vi "ReadIO.fpga.vi"(10 "x (in)":u32, 11 "Memory In":refnum<k21>="InputMatrix") -> (2 "x (out)":u32)   [LabVIEW 2012]
uses:
  <vilib>/rvi/eio/common/nirviEmuTemplateMethod_errors.vi
  <vilib>/rvi/DataTransferAndStorage/Container/Common/niFpgaContainerExecOnDevCompGetState.vi
  <vilib>/rvi/DataTransferAndStorage/Container/Common/niFpgaContainerGetUniqueNameForEmu.vi
  <vilib>/rvi/Memory/Memory_Emulation/niFpgaMemoryEmulationCacheClearOnFirstRun.vi
  <vilib>/rvi/Memory/Memory_Emulation/nirvimemoryEmulationManagerCache_MakeExclusive.vi
  <vilib>/rvi/Memory/Memory_Emulation/niFpgaMemoryEmulationValidateCache.vi
  <vilib>/rvi/Memory/Memory_Emulation/nirvimemoryEmulationManagerCache_ReleaseExclusive.vi
  <vilib>/rvi/Memory/Memory_Emulation/nirvimemoryEmulationManagerCache_InsertValue.vi
  <vilib>/Utility/error.llb/Clear Errors.vi
  <vilib>/rvi/Emulation/niFpgaSctlEmulationGetInTimedLoop.vi
  <vilib>/rvi/Memory/Memory_Emulation/nirvimemoryEmulationManagerCache_GetValue.vi
  <vilib>/rvi/Memory/Memory_Emulation/nirvimemoryEmulationManagerCache_SetValue.vi
  <vilib>/rvi/Emulation/niFpgaSctlEmulationResourceMgr.vi
  <vilib>/eio/EIONode/EIONode.xnode
  <vilib>/rvi/DataTransferAndStorage/Container/XNode/niFpgaContainer.xnode
  <vilib>/rvi/Memory/Memory_Emulation/niFpgaMemoryEmulationRefIn.vi
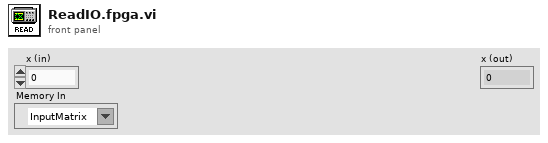
[diagram p1: front panel]
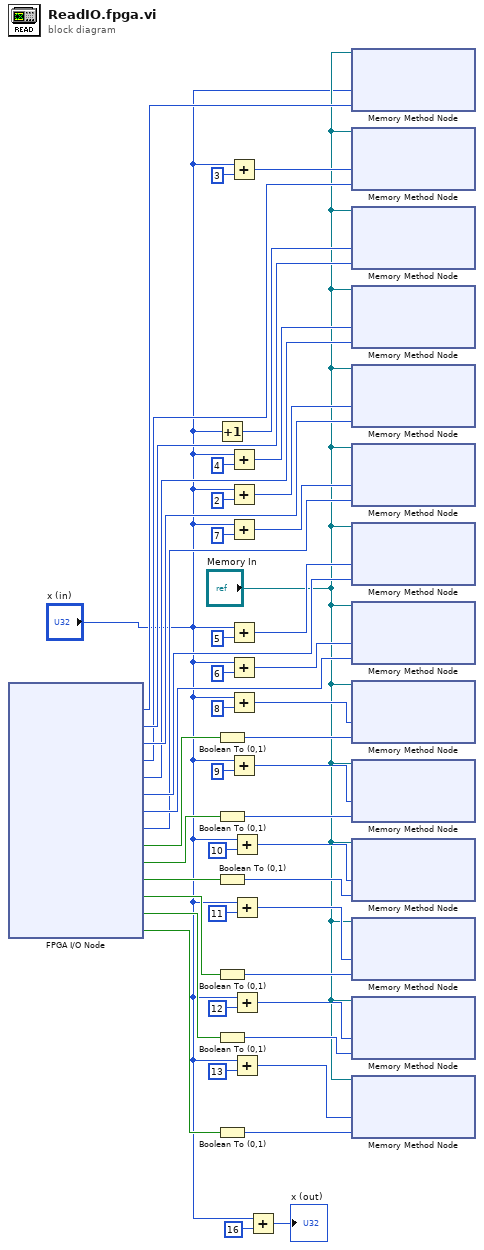
[diagram p0: block diagram]
diagram:
  n1 = xnode "FPGA I/O Node"() -> ("Connector0/AI0"=w49:i16, "Connector0/AI1"=w47:i16, "Connector0/AI2"=w46:i16, "Connector0/AI3"=w45:i16, "Connector0/AI4"=w44:i16, "Connector0/AI5"=w43:i16, "Connector0/AI6"=w42:i16, "Connector0/AI7"=w41:i16, "Connector0/DIO6"=w40:bool, "Connector0/DIO7"=w38:bool, "Connector0/DIO8"=w36:bool, "Connector0/DIO9"=w34:bool, "Connector0/DIO10"=w32:bool, "Connector0/DIO11"=w30:bool)  [unwired: 14 in, 14 out]
  n2 = Increment(x="x (in)") -> (x+1=w48:u32)
  n3 = Boolean To (0,1)(Boolean=w40) -> (0, 1=w39:i16)
  n4 = Boolean To (0,1)(Boolean=w38) -> (0, 1=w37:i16)
  n5 = Boolean To (0,1)(Boolean=w36) -> (0, 1=w35:i16)
  n6 = Boolean To (0,1)(Boolean=w34) -> (0, 1=w33:i16)
  n7 = Boolean To (0,1)(Boolean=w32) -> (0, 1=w31:i16)
  n8 = Boolean To (0,1)(Boolean=w30) -> (0, 1=w29:i16)
  n9 = Add(x="x (in)", y=u32 3) -> (x+y=w25:u32)
  n10 = Add(x="x (in)", y=u32 4) -> (x+y=w23:u32)
  n11 = Add(x="x (in)", y=u32 2) -> (x+y=w27:u32)
  n12 = Add(x="x (in)", y=u32 7) -> (x+y=w17:u32)
  n13 = Add(x="x (in)", y=u32 5) -> (x+y=w21:u32)
  n14 = Add(x="x (in)", y=u32 6) -> (x+y=w19:u32)
  n15 = Add(x="x (in)", y=u32 8) -> (x+y=w15:u32)
  n16 = Add(x="x (in)", y=u32 9) -> (x+y=w13:u32)
  n17 = Add(x="x (in)", y=u32 10) -> (x+y=w11:u32)
  n18 = Add(x="x (in)", y=u32 11) -> (x+y=w9:u32)
  n19 = Add(x="x (in)", y=u32 12) -> (x+y=w7:u32)
  n20 = Add(x="x (in)", y=u32 13) -> (x+y=w5:u32)
  n21 = Add(x="x (in)", y=u32 16) -> (x+y=→"x (out)":u32)
  n22 = xnode ("Memory Method Node")("Address"="x (in)", "Data"=w49, "Memory In"="Memory In") -> ()  [unwired: 1 out]
  n23 = xnode ("Memory Method Node")("Address"=w25, "Data"=w45, "Memory In"="Memory In") -> ()  [unwired: 1 out]
  n24 = xnode ("Memory Method Node")("Address"=w48, "Data"=w47, "Memory In"="Memory In") -> ()  [unwired: 1 out]
  n25 = xnode ("Memory Method Node")("Address"=w23, "Data"=w44, "Memory In"="Memory In") -> ()  [unwired: 1 out]
  n26 = xnode ("Memory Method Node")("Address"=w27, "Data"=w46, "Memory In"="Memory In") -> ()  [unwired: 1 out]
  n27 = xnode ("Memory Method Node")("Address"=w17, "Data"=w41, "Memory In"="Memory In") -> ()  [unwired: 1 out]
  n28 = xnode ("Memory Method Node")("Address"=w21, "Data"=w43, "Memory In"="Memory In") -> ()  [unwired: 1 out]
  n29 = xnode ("Memory Method Node")("Address"=w19, "Data"=w42, "Memory In"="Memory In") -> ()  [unwired: 1 out]
  n30 = xnode ("Memory Method Node")("Address"=w15, "Data"=w39, "Memory In"="Memory In") -> ()  [unwired: 1 out]
  n31 = xnode ("Memory Method Node")("Address"=w13, "Data"=w37, "Memory In"="Memory In") -> ()  [unwired: 1 out]
  n32 = xnode ("Memory Method Node")("Address"=w11, "Data"=w35, "Memory In"="Memory In") -> ()  [unwired: 1 out]
  n33 = xnode ("Memory Method Node")("Address"=w9, "Data"=w33, "Memory In"="Memory In") -> ()  [unwired: 1 out]
  n34 = xnode ("Memory Method Node")("Address"=w7, "Data"=w31, "Memory In"="Memory In") -> ()  [unwired: 1 out]
  n35 = xnode ("Memory Method Node")("Address"=w5, "Data"=w29, "Memory In"="Memory In") -> ()  [unwired: 1 out]
